vi "Close Cal Standard If Necessary.vi"(11 "error in (no error)":errorcluster) -> (15 "error out":errorcluster)   [LabVIEW 2023, in "RFFixtureCharact.Instruments.lvlib" / "Cal Standard Factory.lvclass"]
uses:
  Cal Standard Factory.lvclass
  Cal Standard Base/Cal Standard Base.lvclass
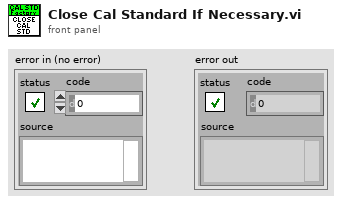
[diagram p1: front panel]
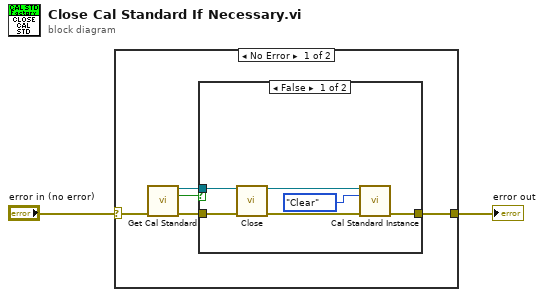
[diagram p0: block diagram]
diagram:
  n1 = case shown="No Error" "error in (no error)" {
    selector: "error in (no error)" -> [w6 w15]
    tunnel: [w7 w15] -> w1
    frame No Error {
      n2 = call "Get Cal Standard.vi"("error in (no error)"=w6) -> ("Cal Standard Base out"=w4:refnum<class "Cal Standard Base.lvclass">, "Not found"=w3:bool, "error out"=w5:errorcluster)  [unwired: 12 in]
      n3 = case shown="False" w3 {
        tunnel: w5 -> [w11 w14]
        tunnel: [w12 w14] -> w7
        tunnel: w4 -> [w10 _]
        frame False {
          n4 = call-dynamic "Close.vi"("Cal Standard Base in"=w10, "error in (no error)"=w11) -> ("Cal Standard Base out"=w8:refnum<class "Cal Standard Base.lvclass">, "error out"=w13:errorcluster)  [unwired: 12 in]
          n5 = call "Cal Standard Instance.vi"("Cal Standard Base in"=w8, "Operation"=enum16{"Read", "Write", "Clear"}."Clear", "error in (no error)"=w13) -> ("error out"=w12:errorcluster)  [unwired: 10 in, 2 out]
        }
        frame True {
        }
      }
    }
    frame Error {
    }
  }
  "error out" <- w1
